vi "Save-Recall Instrument Setup from file.vi"(0 "VISA resource name":refnum<visa-resource-name>, 5 "Action (0:Save Instrument Setup)":u16(ring) items=["Save Instrument Setup", "Recall Instrument Setup"], 9 "Timeout":u32=10000, 11 "error in (no error)":errorcluster, 12 "Path (D:\\Setups)":string="D:\\Setups", 13 "Filename (panel.lss)":string="panel.lss") -> (4 "VISA resource name out":refnum<visa-resource-name>, 15 "error out":errorcluster)   [LabVIEW 2015, in "LeCroy Wave Series.lvlib"]
doc: "Stores/Recall the current state of your instrument to/from a file on the scope's harddrive.\n\nTo save or recall panel setups to one of the \"internal\" non-volatile memories, use the VI \"Save-Recall Setup\""
uses:
  <instrlib>/LeCroy Wave Series/LeCroy Wave Series.lvlib
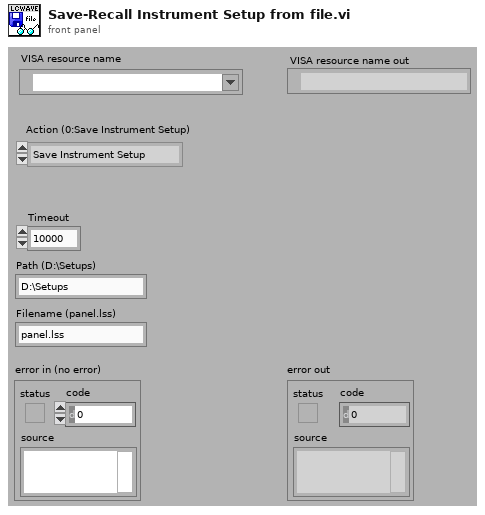
[diagram p1: front panel]
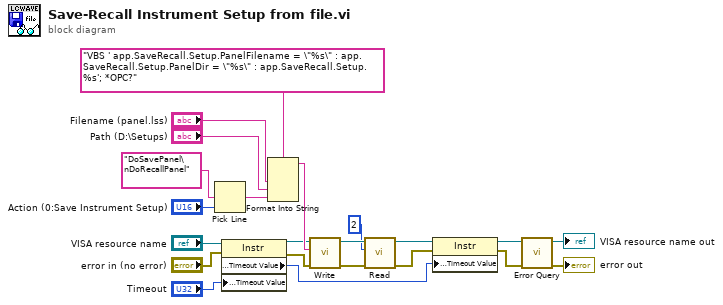
[diagram p0: block diagram]
diagram:
  n1 = Pick Line(multi-line string="DoSavePanel\nDoRecallPanel", line index="Action (0:Save Instrument Setup)") -> (output string=w3:string)  [unwired: 1 in]
  n2 = property class="Instr"(reference="VISA resource name", error in="error in (no error)", "General Settings:Timeout Value"="Timeout") -> (reference out=w13:refnum<visa-resource-name>, error out=w7:errorcluster, "General Settings:Timeout Value"=w6:u32)
  n3 = Format Into String(format string="VBS ' app.SaveRecall.Setup.PanelFilename = \"%s\" : app.SaveRecall.Setup.PanelDir = \"%s\" : app.SaveRecall.Setup.%s'; *OPC?", "Filename (panel.lss)", "Path (D:\\Setups)", w3) -> (resulting string=w20:string)  [unwired: 2 in, 1 out]
  n4 = call <instrlib>:"Write.vi"("error in (no error)"=w7, "Write Buffer"=w20, "VISA resource name"=w13) -> ("error out"=w15:errorcluster, "VISA resource name out"=w16:refnum<visa-resource-name>)  [unwired: 6 in, 1 out]
  n5 = call <instrlib>:"Read.vi"("error in (no error)"=w15, "Byte Count"=u32 2, "VISA resource name"=w16) -> ("error out"=w2:errorcluster, "VISA resource name out"=w11:refnum<visa-resource-name>)  [unwired: 5 in, 2 out]
  n6 = property class="Instr"(reference=w11, error in=w2, "General Settings:Timeout Value"=w6) -> (reference out=w12:refnum<visa-resource-name>, error out=w1:errorcluster)
  n7 = call <instrlib>:"Error Query.vi"("error in (no error)"=w1, "VISA resource name"=w12) -> ("error out"=→"error out":errorcluster, "VISA resource name out"=→"VISA resource name out":refnum<visa-resource-name>)  [unwired: 6 in, 2 out]
